vi "execute_initial_value_policy.vi"(8 "error in (no error)":errorcluster, 9 "Last Publish Time":timestamp, 10 "Last Topic Value":variant, 11 "BasicSubscription In":refnum<class "BasicSubscription.lvclass">) -> (0 "error out":errorcluster, 3 "BasicSubscription Out":refnum<class "BasicSubscription.lvclass">)   [LabVIEW 2017, in "SubscriptionPolicy.lvlib" / "BasicSubscription.lvclass"]
uses:
  BasicSubscription.lvclass
  C:/Git/mva-framework/Framework/IMediator/ISubscriptionPolicy/ISubscriptionPolicy.lvclass
  BasicSubscription.lvclass/BasicSubscription.ctl
  IMediator/ISubscriptionPolicy/ISubscriptionPolicy.lvclass/ISubscriptionPolicy.ctl
  IMediator/ITransport/ITransport.lvclass
  IMediator/ISubscriptionPolicy/ISubscriptionPolicy.lvclass
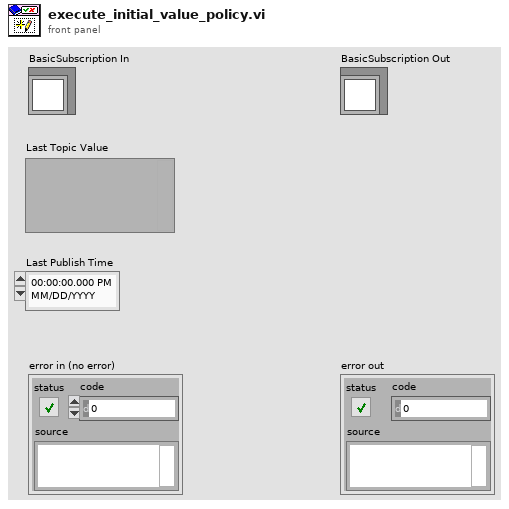
[diagram p1: front panel]
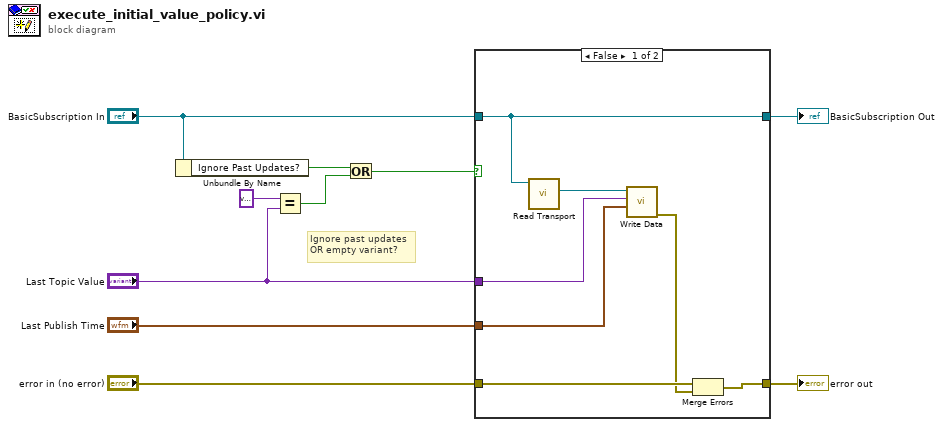
[diagram p0: block diagram]
diagram:
  # "Ignore past updates\nOR empty variant?"
  n1 = Unbundle By Name("BasicSubscription In") -> ("Ignore Past Updates?"=w3:bool)
  n2 = Equal?(x=variant, y="Last Topic Value") -> (x = y?=w4:bool)
  n3 = Or(x=w3, y=w4) -> (x .or. y?=w2:bool)
  n4 = case shown="False" w2 {
    tunnel: "error in (no error)" -> [w17 w18]
    tunnel: "Last Topic Value" -> [w16 _]
    tunnel: "Last Publish Time" -> [w15 _]
    tunnel: [w14 w18] -> w8
    tunnel: "BasicSubscription In" -> [w11 w19]
    tunnel: [w11 w19] -> w7
    frame False {
      n5 = call "Read Transport.vi"("ISubscriptionPolicy in"=w11) -> ("Transport"=w12:refnum<class "ITransport.lvclass">)  [unwired: 10 in]
      n6 = call-dynamic "Write Data.vi"("Publication Time"=w15, "Value"=w16, "ITransport in"=w12) -> ("error out"=w13:errorcluster)  [unwired: 7 in, 1 out]
      n7 = Merge Errors(w17, w13) -> (w14:errorcluster)
    }
    frame True {
    }
  }
  "error out" <- w8
  "BasicSubscription Out" <- w7
